vi "Wood Inspection.vi"() -> ()   [LabVIEW 2017]
doc: "Printed Circuit Board Inspection\nDetermine whether PCB components are present and in the correct location using pattern matching. Match areas of inspection to a template of valid components. Use shift-invariant matching to inspect an oriented component (diode). Use rotation-invariant matching to inspect an unoriented component (resistor)."
uses:
  IMAQCV/IMAQCV.lvlib
  IMAQCV/LVOpenCV.lvlib
panel:
  in  "Image Delay ms":u32=5000
  out "Image":T1(plugin-control)
  in  "Image File path":path=path "c:/vision/Wood/Wood1.jpg"
  out "Image Log path":path=path "c:/vision/Result.jpg"
  out "error out":errorcluster
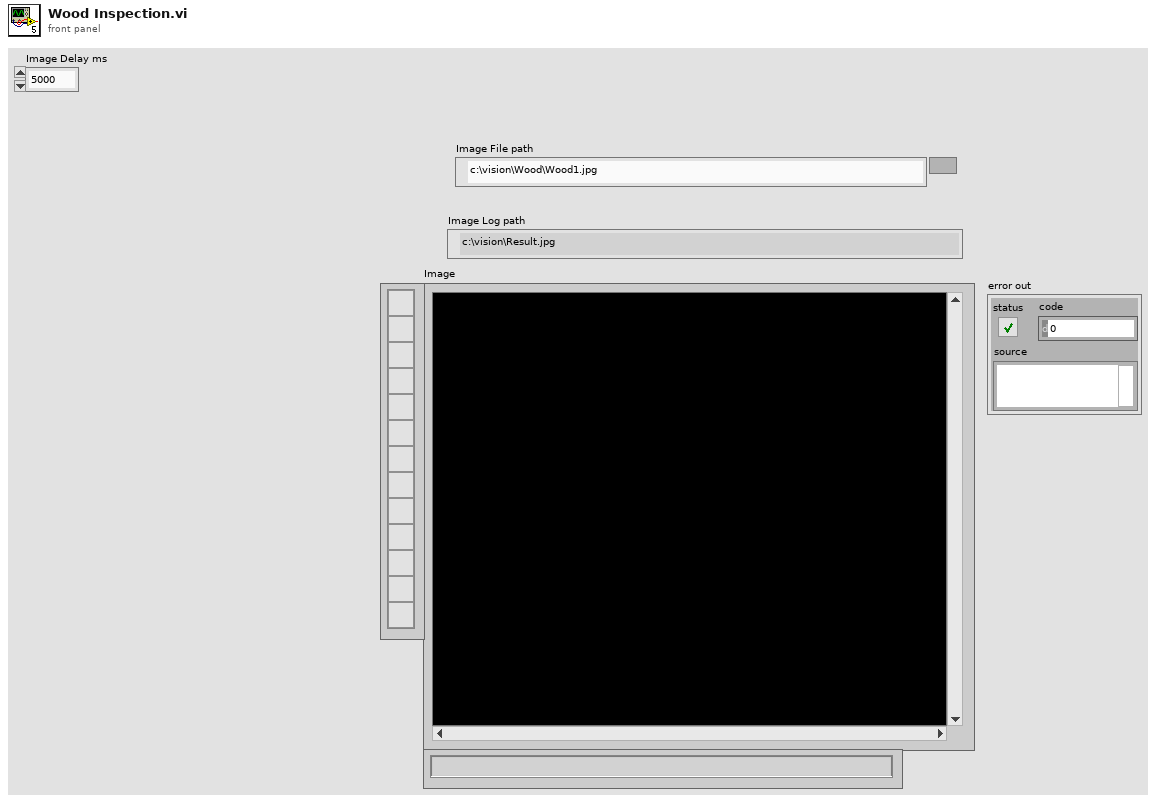
[diagram p1: front panel]
types:
  T1 = typedef "IMAQ Image.ctl" = refnum<image>
  T2 = typedef "Image Type" = u32
  T3 = typedef "IMAQCV.lvlib/IMAQCV Image.ctl" = refnum<vi>
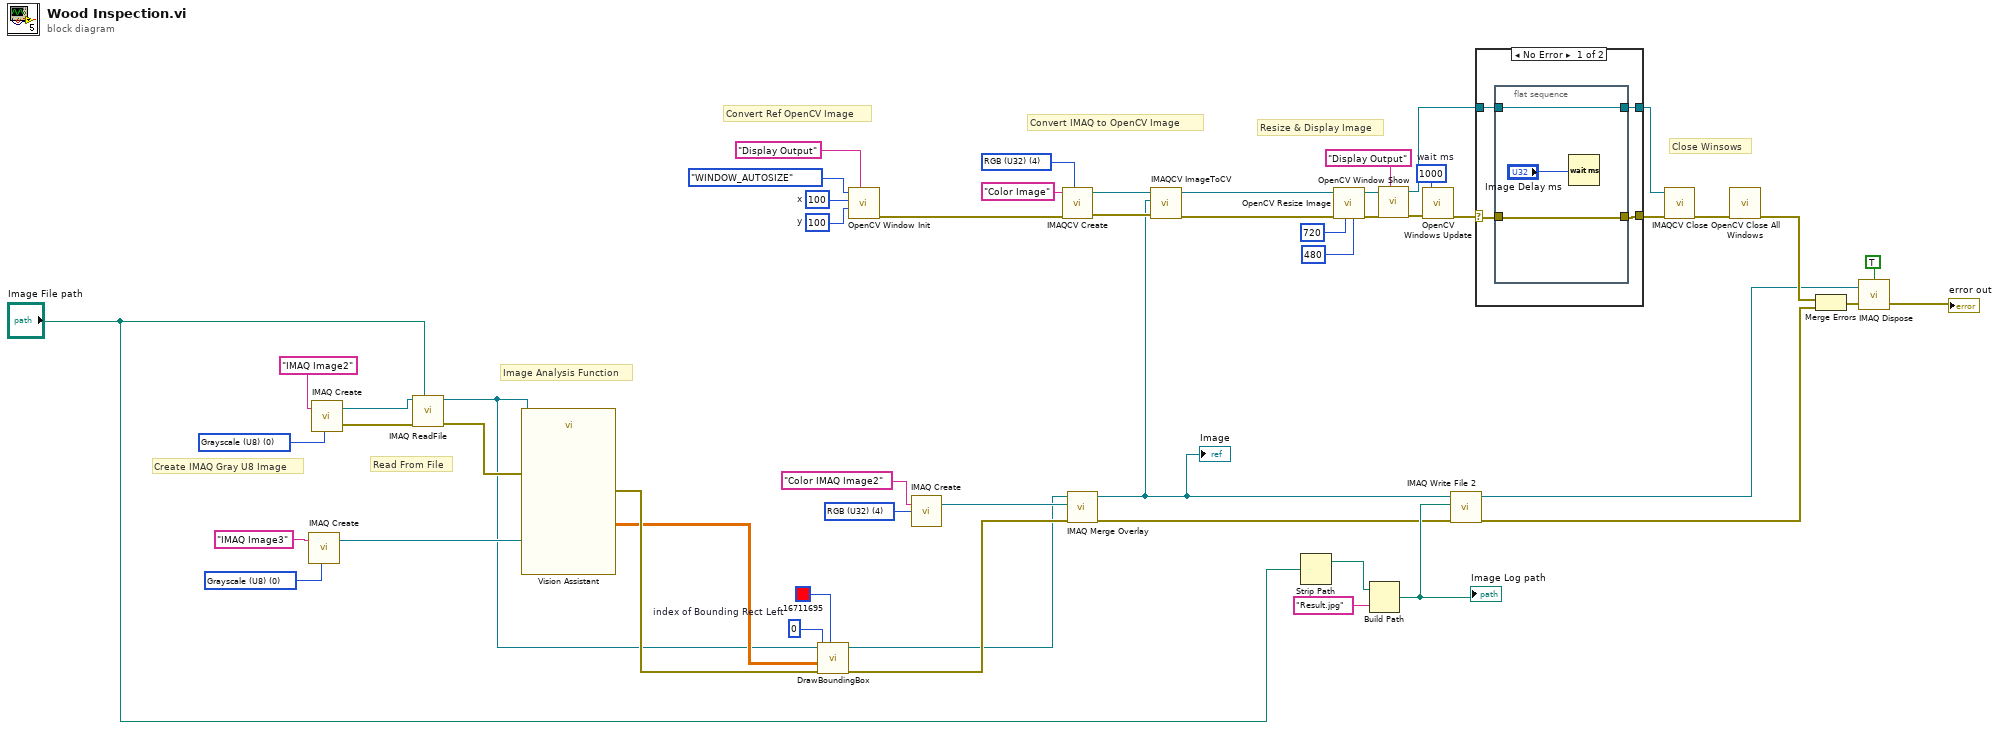
[diagram p0: block diagram]
diagram:
  w18 = 1000  # wait ms
  w25 = u32 100  # y
  w26 = u32 100  # x
  w29 = u32 4 items=["Grayscale (U8)", "Grayscale (I16)", "Grayscale (SGL)", "Complex (CSG)", "RGB (U32)", "HSL (U32)", "RGB (U64)", "Grayscale (U16)"] ("Image Type")
  w34 = T2 0 items=["Grayscale (U8)", "Grayscale (I16)", "Grayscale (SGL)", "Complex (CSG)", "RGB (U32)", "HSL (U32)", "RGB (U64)", "Grayscale (U16)"] ("Image Type")
  w41 = 0  # index of Bounding Rect Left
  w48 = T2 4 items=["Grayscale (U8)", "Grayscale (I16)", "Grayscale (SGL)", "Complex (CSG)", "RGB (U32)", "HSL (U32)", "RGB (U64)", "Grayscale (U16)"] ("Image Type")
  w2 = T2 0 items=["Grayscale (U8)", "Grayscale (I16)", "Grayscale (SGL)", "Complex (CSG)", "RGB (U32)", "HSL (U32)", "RGB (U64)", "Grayscale (U16)"] ("Image Type")
  # "Close Winsows"
  # "Resize & Display Image"
  # "Convert Ref OpenCV Image"
  # "Convert IMAQ to OpenCV Image"
  # "Image Analysis Function"
  # "Read From File"
  # "Create IMAQ Gray U8 Image"
  n1 = call "IMAQ Create"("Image Name"="IMAQ Image3", "Image Type"=w34) -> ("New Image"=w35:T1)  [unwired: 2 in, 2 out]
  n2 = call "IMAQ Create"("Image Name"="IMAQ Image2", "Image Type"=w2) -> ("New Image"=w52:T1, "error out"=w51:errorcluster)  [unwired: 2 in, 1 out]
  n3 = call "IMAQ ReadFile"("File Path"="Image File path", "error in (no error)"=w51, "Image"=w52) -> ("error out"=w50:errorcluster, "Image Out"=w32:T1)  [unwired: 2 in, 5 out]
  n4 = call "Vision Assistant"("Image In"=w32, "Image Dst"=w35, "error in"=w50) -> ("Particle Measurements (Pixels) (Particle Analysis 1)"=w38:dbl[][], "error out"=w39:errorcluster)  [unwired: 21 in, 2 out]
  n5 = call "DrawBoundingBox.vi"("Color"=u32 16711695, "error in (no error)"=w39, "Particle Measurements"=w38, "index of Bounding Rect Left"=w41, "Image"=w32) -> ("error out"=w37:errorcluster, "Image 2"=w33:T1)  [unwired: 5 in]
  n6 = call "OpenCV Window Init.vi"("window name"="Display Output", "y"=w25, "x"=w26, "mode"=enum8{"WINDOW_AUTOSIZE", "WINDOW_FULLSCREEN"}."WINDOW_AUTOSIZE") -> ("error out"=w9:errorcluster)  [unwired: 7 in]
  n7 = call "IMAQ Create"("Image Name"="Color IMAQ Image2", "Image Type"=w48) -> ("New Image"=w47:T1)  [unwired: 2 in, 2 out]
  n8 = call "IMAQCV Create.vi"("Image Type"=w29, "error in (no error)"=w9, "Image Name"="Color Image") -> ("error out"=w12:errorcluster, "Image Out"=w30:T3)  [unwired: 7 in]
  n9 = call "IMAQ Merge Overlay"("error in (no error)"=w37, "Image Dst"=w47, "Image Src"=w33) -> ("error out"=w42:errorcluster, "Image Dst Out"=w1:T1)  [unwired: 7 in]
  "Image" <- w1
  n10 = call "IMAQCV ImageToCV.vi"("error in (no error)"=w12, "Variant In"=w1, "CV in"=w30) -> ("error out"=w8:errorcluster, "CV out"=w17:T3)  [unwired: 7 in]
  n11 = Strip Path(path="Image File path") -> (stripped path=w45:path)  [unwired: 1 out]
  n12 = call "OpenCV Resize Image.vi"("height"=u32 480, "width"=u32 720, "error in (no error)"=w8, "image in"=w17) -> ("error out"=w21:errorcluster, "image out"=w22:T3)  [unwired: 6 in]
  n13 = Build Path(base path=w45, name or relative path="Result.jpg") -> (appended path=w43:path)
  "Image Log path" <- w43
  n14 = call "OpenCV Window Show.vi"("window name"="Display Output", "error in (no error)"=w21, "image in"=w22) -> ("error out"=w23:errorcluster, "image out"=w15:T3)  [unwired: 7 in]
  n15 = call "OpenCV Windows Update.vi"("error in (no error)"=w23, "wait ms"=w18) -> ("error out"=w11:errorcluster)  [unwired: 8 in, 1 out]
  n16 = call-poly "IMAQ Write File 2"("error in (no error)"=w42, "File Path"=w43, "Image"=w1) -> ("error out"=w3:errorcluster, "Image Out (duplicate)"=w4:T1)  [unwired: 7 in]
  n17 = case shown="No Error" w11 {
    selector: w11 -> [w54 w62]
    tunnel: [w57 w62] -> w16
    tunnel: w15 -> [w56 w61]
    tunnel: [w55 w61] -> w14
    frame No Error {
      n18 = flat-sequence {
        tunnel: [w60] -> w57
        tunnel: w54 -> [w60]
        tunnel: [w59] -> w55
        tunnel: w56 -> [w59]
        frame #0 {
          n19 = Wait (ms)(milliseconds to wait="Image Delay ms") -> ()  [unwired: 1 out]
        }
      }
    }
    frame Error {
    }
  }
  n20 = call "IMAQCV Close.vi"("error in (no error)"=w16, "Image"=w14) -> ("error out"=w13:errorcluster)  [unwired: 9 in]
  n21 = call "OpenCV Close All Windows.vi"("error in (no error)"=w13) -> ("error out"=w6:errorcluster)  [unwired: 10 in]
  n22 = Merge Errors(w6, w3) -> (w7:errorcluster)
  n23 = call "IMAQ Dispose"("All Images? (No)"=TRUE, "Image"=w4, "error in (no error)"=w7) -> ("error out"=→"error out":errorcluster)  [unwired: 3 in]
